vi "Init.vi"(8 "error in (no error)":errorcluster, 10 "Topic":string, 11 "Pub Sub Retaining Message Channel in":refnum<class "Pub Sub Retaining Message Channel.lvclass">) -> (0 "error out":errorcluster, 3 "Pub Sub Retaining Message Channel out":refnum<class "Pub Sub Retaining Message Channel.lvclass">)   [LabVIEW 2020, in "Actor Pub Sub Channels.lvlib" / "Pub Sub Retaining Message Channel.lvclass"]
uses:
  Pub Sub Retaining Message Channel.lvclass
  <vilib>/ActorFramework/Message/Message.lvclass
  Pub Sub Retaining Message Channel.lvclass/Pub Sub Retaining Message Channel.ctl
  Pub Sub Message Channel/Pub Sub Message Channel.lvclass
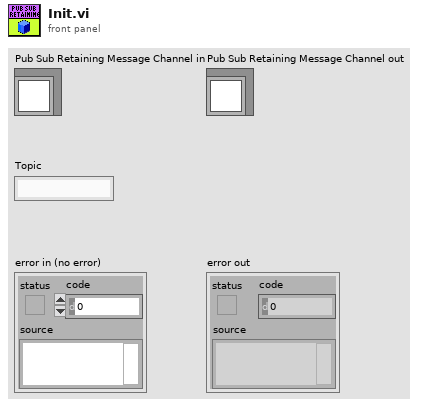
[diagram p1: front panel]
types:
  T1 = cluster{"Actor Framework:Message":refnum<class "Message.lvclass">}
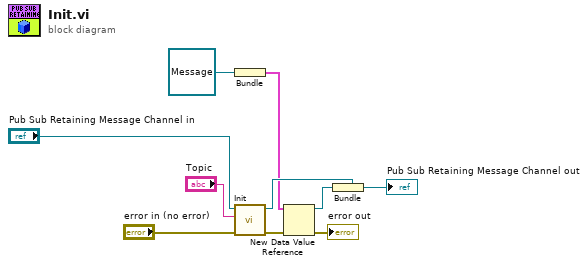
[diagram p0: block diagram]
diagram:
  n1 = Bundle("Actor Framework:Message"=refnum<class "Message.lvclass"> refnum) -> (w5:T1)  [unwired: 1 in]
  n2 = call-parent "Init.vi"("error in (no error)"="error in (no error)", "Topic"="Topic", "Pub Sub Message Channel in"="Pub Sub Retaining Message Channel in") -> ("error out"=w2:errorcluster, "Pub Sub Message Channel out"=w10:refnum<class "Pub Sub Retaining Message Channel.lvclass">)  [unwired: 7 in]
  n3 = New Data Value Reference(data value=w5, error in=w2) -> (data value reference=w3:refnum<data-value>, error out=→"error out":errorcluster)
  n4 = Bundle(cluster=w10, w3) -> (→"Pub Sub Retaining Message Channel out":refnum<class "Pub Sub Retaining Message Channel.lvclass">)
